vi "数据长度修改.vi"   [LabVIEW 2013]
uses:
  <vilib>/Utility/file.llb/Read From Spreadsheet File (I64).vi
  <vilib>/Utility/file.llb/Write To Spreadsheet File (I64).vi
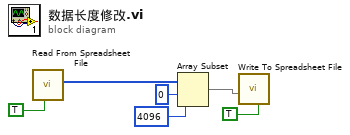
[diagram p0: block diagram]
diagram:
  n1 = call-poly <vilib>:"Read From Spreadsheet File.vi"("transpose (no:F)"=TRUE) -> ("first row"=w6:i64[])  [unwired: 6 in, 4 out]
  n2 = Array Subset(array=w6, index=0 ("索引"), length=4096 ("长度")) -> (w3:i64[])
  n3 = call-poly <vilib>:"Write To Spreadsheet File.vi"("transpose? (no:F)"=TRUE, "1D data"=w3) -> ()  [unwired: 6 in, 1 out]
